vi "Set Server gRPC UEs.vi"(10 "Server gRPC UEs":T1, 11 "OOP Server in":refnum<class "TestServer.lvclass">) -> (3 "OOP Server out":refnum<class "TestServer.lvclass">)   [LabVIEW 2019, in "TestServer.lvlib" / "TestServer.lvclass"]
uses:
  TestServer.lvclass
  typeDefs/Server gRPC UEs.ctl
  gRPC lvSupport/Server API/typeDefs/gRPCId Cluster.ctl
  gRPC lvSupport/Server API/typeDefs/grpcId.ctl
  TestServer.lvclass/TestServer.ctl
  gRPC lvSupport/gprc-lvsupport.lvlib
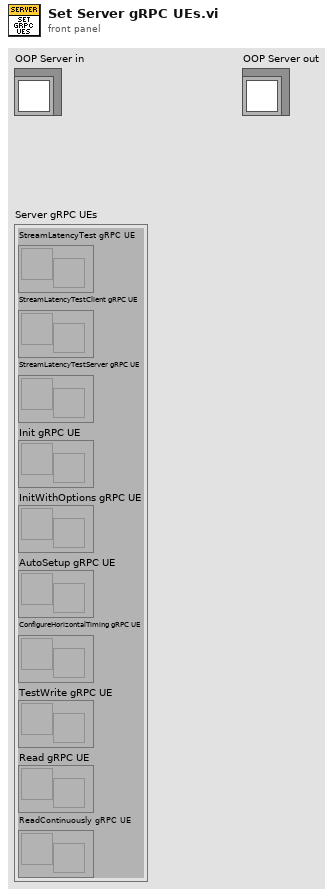
[diagram p1: front panel]
types:
  T1 = typedef "TestServer.lvlib/TestServer.lvclass/Server gRPC UEs.ctl" = cluster{"StreamLatencyTest gRPC UE":refnum<user-event>, "StreamLatencyTestClient gRPC UE":refnum<user-event>, "StreamLatencyTestServer gRPC UE":refnum<user-event>, "Init gRPC UE":refnum<user-event>, "InitWithOptions gRPC UE":refnum<user-event>, "AutoSetup gRPC UE":refnum<user-event>, "ConfigureHorizontalTiming gRPC UE":refnum<user-event>, "TestWrite gRPC UE":refnum<user-event>, "Read gRPC UE":refnum<user-event>, "ReadContinuously gRPC UE":refnum<user-event>}
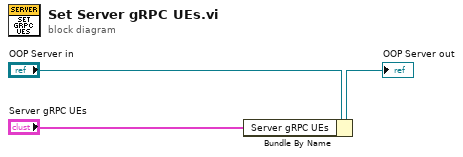
[diagram p0: block diagram]
diagram:
  n1 = Bundle By Name(cluster="OOP Server in", "Server gRPC UEs"="Server gRPC UEs") -> (→"OOP Server out":refnum<class "TestServer.lvclass">)
